vi "XMLTags.vi"() -> (0 "<Val>":string, 5 "</Val>":string, 6 "<Version>":string, 7 "</Version>":string, 8 "<Object>":string, 9 "</Object>":string, 10 "<Name>":string, 11 "</Name>":string, 12 "<Type>":string, 13 "</Type>":string, 14 "<Class>":string, 15 "<PrivateData>":string, 16 "</PrivateData>":string, 17 "<ClassVariable>":string, 18 "</ClassVariable>":string, 19 "</Class>":string)   [LabVIEW 2020, in "OpenG_Object.lvclass"]
doc: "Specifies a set of XML tags to be used for converting objects to XML and for creating objects from XML."
uses:
  OpenG_Object.lvclass
panel:
  # "Please visit http://www.OpenG.org to learn about the\nOpen Source LabVIEW software movement.\n\nNOTICE -- YOU MUST LEAVE THIS NOTICE IN PLACE.  PER THE TERMS OF THE LICENSE BELOW, YOU MAY SUBLICENSE THIS SOFTWARE \nIN ANY WAY THAT DOES NOT CONFLICT WITH THIS LICENSE.\n\n### BSD License (http://www.opensource.org/licenses/bsd-license.php) Begin ###\n\nCopyright (c) 2007, Tomi Maila\nCopyright (c) 2007, Endevo AB\n\n\nAll rights reserved.\n\nRedistribution and use in source and binary forms, with or without modification, are permitted provided that the following conditions are met:\n\n    * Redistributions of source code must retain the above copyright notice, this list of conditions and the following disclaimer.\n    * Redistributions in binary form must reproduce the above copyright notice, this list of conditions and the following disclaimer in the \n       documentation and/or other materials provided with the distribution.\n    * Neither the name of Endevo AB nor the names of the contributors may be used to endorse or promote products derived\n       from this software without specific prior written permission.\n\nTHIS SOFTWARE IS PROVIDED BY THE COPYRIGHT HOLDERS AND CONTRIBUTORS \"AS IS\" AND ANY EXPRESS OR IMPLIED WARRANTIES, \nINCLUDING, BUT NOT LIMITED TO, THE IMPLIED WARRANTIES OF MERCHANTABILITY AND FITNESS FOR A PARTICULAR PURPOSE ARE \nDISCLAIMED. IN NO EVENT SHALL THE COPYRIGHT OWNER OR CONTRIBUTORS BE LIABLE FOR ANY DIRECT, INDIRECT, INCIDENTAL,\n SPECIAL, EXEMPLARY, OR CONSEQUENTIAL DAMAGES (INCLUDING, BUT NOT LIMITED TO, PROCUREMENT OF SUBSTITUTE GOODS OR \nSERVICES; LOSS OF USE, DATA, OR PROFITS; OR BUSINESS INTERRUPTION) HOWEVER CAUSED AND ON ANY THEORY OF LIABILITY, \nWHETHER IN CONTRACT, STRICT LIABILITY, OR TORT (INCLUDING NEGLIGENCE OR OTHERWISE) ARISING IN ANY WAY OUT OF THE USE \nOF THIS SOFTWARE, EVEN IF ADVISED OF THE POSSIBILITY OF SUCH DAMAGE.\n\n### BSD License End ###"
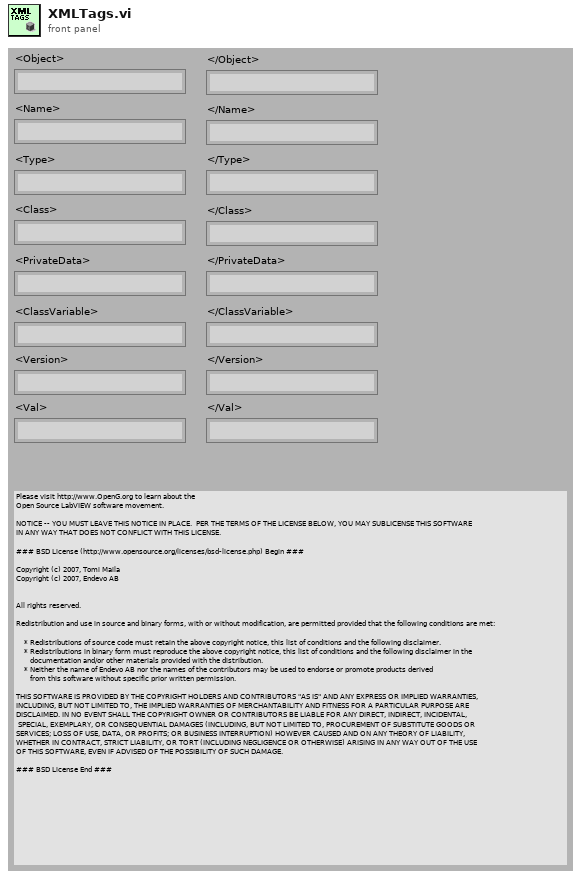
[diagram p1: front panel]
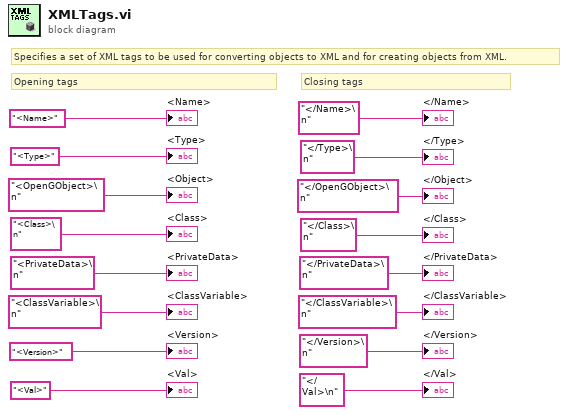
[diagram p0: block diagram]
diagram:
  # "Closing tags"
  # "Opening tags"
  # "Specifies a set of XML tags to be used for converting objects to XML and for creating objects from XML."
  "<Object>" <- "<OpenGObject>\n" ("Begin")
  "</Object>" <- "</OpenGObject>\n" ("Begin")
  "<Class>" <- "<Class>\n" ("Begin")
  "</Class>" <- "</Class>\n" ("Begin")
  "<Type>" <- "<Type>" ("<Type>")
  "</Type>" <- "</Type>\n" ("</Type>")
  "<PrivateData>" <- "<PrivateData>\n" ("<PrivateData>")
  "</PrivateData>" <- "</PrivateData>\n" ("</PrivateData>")
  "<ClassVariable>" <- "<ClassVariable>\n" ("<ClassData>")
  "</ClassVariable>" <- "</ClassVariable>\n" ("</ClassData>")
  "<Name>" <- "<Name>" ("<Name>")
  "</Name>" <- "</Name>\n" ("</Name>")
  "<Version>" <- "<Version>" ("<Version>")
  "</Version>" <- "</Version>\n" ("</Version>")
  "<Val>" <- "<Val>" ("<Val>")
  "</Val>" <- "</Val>\n" ("</Val>")
